vi "command wait for stop.vi"(8 "error in (no error)":errorcluster, 10 "refresh_interval_ms":u32, 11 "id":i32) -> (0 "error out":errorcluster, 3 "function return":i32)   [LabVIEW 2012, in "libximc.lvlib"]
doc: "result_t XIMC_API command_wait_for_stop(device_t id, uint32_t refresh_interval_ms);"
uses:
  libximc.lvlib
  libximc.dll
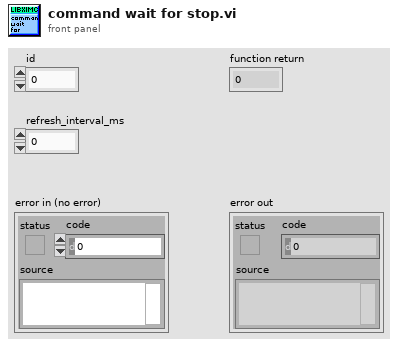
[diagram p1: front panel]
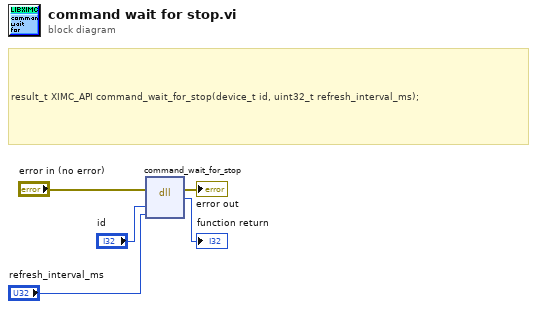
[diagram p0: block diagram]
diagram:
  # "result_t XIMC_API command_wait_for_stop(device_t id, uint32_t refresh_interval_ms);"
  n1 = dll-call lib="C:/Users/Vasily/Att_examples/LabVIEW_example/libximc.*" fn="command_wait_for_stop"(error in="error in (no error)", "id"="id", "refresh_interval_ms"="refresh_interval_ms") -> (error out=→"error out":errorcluster, →"function return":i32)  [unwired: 4 in, 1 out]
